vi "Get Measurements.vi"(10 "Setpoint":dbl) -> (2 "Linear Actuator Length":dbl=16.250611653573802, 3 "Length":dbl=54.82928049865327)   [LabVIEW 2017]
panel:
  in  "h":dbl=21.75
  in  "hinge to boundary":dbl=23.0 format="%#_13g"
  out "Angle":dbl=0.8176450458327023
  in  "Constant":dbl=12.25
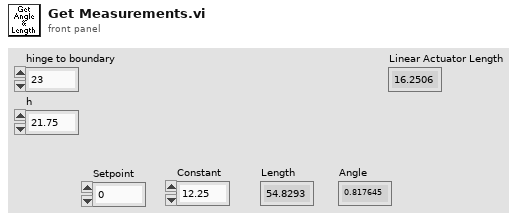
[diagram p1: front panel]
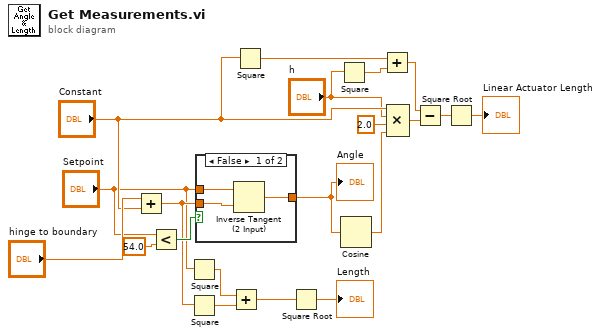
[diagram p0: block diagram]
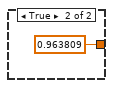
[diagram p2: hidden frame]
diagram:
  n1 = Add(x="hinge to boundary", y="Constant") -> (x+y=w3:dbl)
  n2 = Less?(x="Setpoint", y=54.0) -> (x < y?=w4:bool)
  n3 = Square(x="Setpoint") -> (x^2=w18:dbl)
  n4 = Square(x=w3) -> (x^2=w19:dbl)
  n5 = case shown="False" w4 {
    tunnel: w3 -> [w23 _]
    tunnel: "Setpoint" -> [w22 _]
    tunnel: [w21 0.963809] -> w1
    frame False {
      n6 = Inverse Tangent (2 Input)(1:w23, 2:w22) -> (0:w21:dbl)
    }
    frame True {
    }
  }
  "Angle" <- w1
  n7 = Add(x=w18, y=w19) -> (x+y=w20:dbl)
  n8 = Square(x="Constant") -> (x^2=w15:dbl)
  n9 = Square Root(x=w20) -> (sqrt(x)=→"Length":dbl)
  n10 = Square(x="h") -> (x^2=w14:dbl)
  n11 = Cosine(x=w1) -> (cos(x)=w10:dbl)
  n12 = Add(x=w15, y=w14) -> (x+y=w9:dbl)
  n13 = Compound Arithmetic op=MULTIPLY("Constant", "h", 2.0 ("value"), w10) -> (w8:dbl)
  n14 = Subtract(x=w9, y=w8) -> (x-y=w7:dbl)
  n15 = Square Root(x=w7) -> (sqrt(x)=→"Linear Actuator Length":dbl)
